vi "Cauchy Random.vi"(6 "seed":i32=-1, 7 "reset":bool, 9 "b":dbl=2.0, 10 "a":dbl=1.0, 11 "samples":i32=128) -> (0 "error":i32, 3 "Cauchy random data":dbl[](array[numeric]))   [LabVIEW 2020, in "NI_Gmath.lvlib"]
doc: "Generates random values from a variate X, where X describes the selected distribution type. You must manually select the polymorphic instance to use."
uses:
  NI_Gmath.lvlib
  st_error_code.ctl
panel:
  # "Cauchy Random"
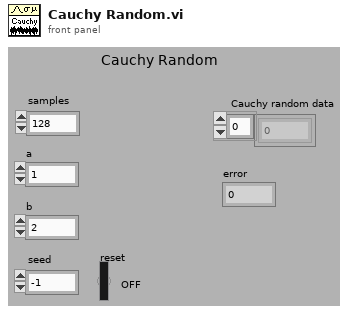
[diagram p1: front panel]
types:
  T1 = typedef "NI_Gmath.lvlib/st_error_code.ctl" = i32
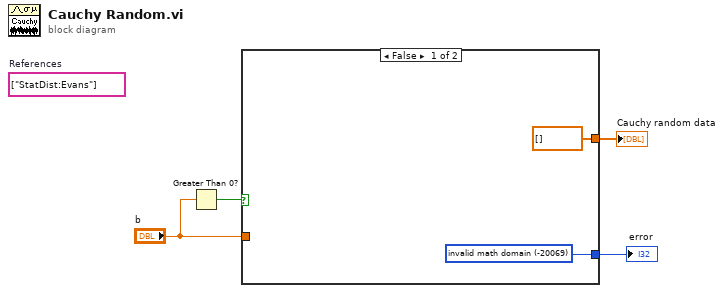
[diagram p0: block diagram]
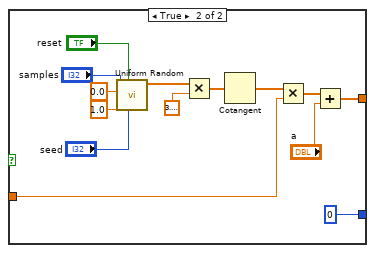
[diagram p2: hidden frame]
diagram:
  (unwired) string[] ["StatDist:Evans"]  # References
  n1 = Greater Than 0?(x="b") -> (x > 0?=w1:bool)
  n2 = case shown="False" w1 {
    tunnel: [dbl[] [] w9] -> w4
    tunnel: "b" -> [_ w8]
    tunnel: [w5 0] -> w2
    frame False {
      w5 = T1 -20069 items=["invalid math domain"=-20069, "Fourier interpolation size m >= n"=-20070, "empty array"=-20003] ("stat interp error code")
    }
    frame True {
      n3 = call "Uniform Random.vi"("seed"="seed", "reset"="reset", "xmax"=1.0, "xmin"=0.0, "samples"="samples") -> ("uniform random data"=w10:dbl[])  [unwired: 5 in, 1 out]
      n4 = Multiply(x=w10, y=3.141592653589793) -> (x*y=w14:dbl[])
      n5 = Cotangent(1:w14) -> (0:w13:dbl[])
      n6 = Multiply(x=w13, y=w8) -> (x*y=w12:dbl[])
      n7 = Add(x=w12, y="a") -> (x+y=w9:dbl[])
    }
  }
  "Cauchy random data" <- w4
  "error" <- w2
